vi "Auxiliary Association (Read).vi"(6 "ISOBUS address":T5=-1 caption="ISOBUS address (-1)", 8 "error in":errorcluster, 11 "Mercury Reference In":T2) -> (0 "error out":errorcluster, 2 "Auxiliary board UID":string, 3 "Mercury Reference Out":T2, 4 "Valid?":T1)   [LabVIEW 2014, in "Mercury iXX.lvlib" / "Control Loop.lvlib"]
doc: "Read the UID of the associated auxiliary board to the control loop."
uses:
  Control Loop.lvlib
  Controls/Mercury Reference.ctl
  Controls/Comms Transport Layer.ctl
  Private/Controls/Query Dynamic Reference.ctl
  Controls/ISOBus Address.ctl
  Controls/Is Valid LED.ctl
  Private/Controls/Command Verbs.ctl
  Mercury iXX.lvlib
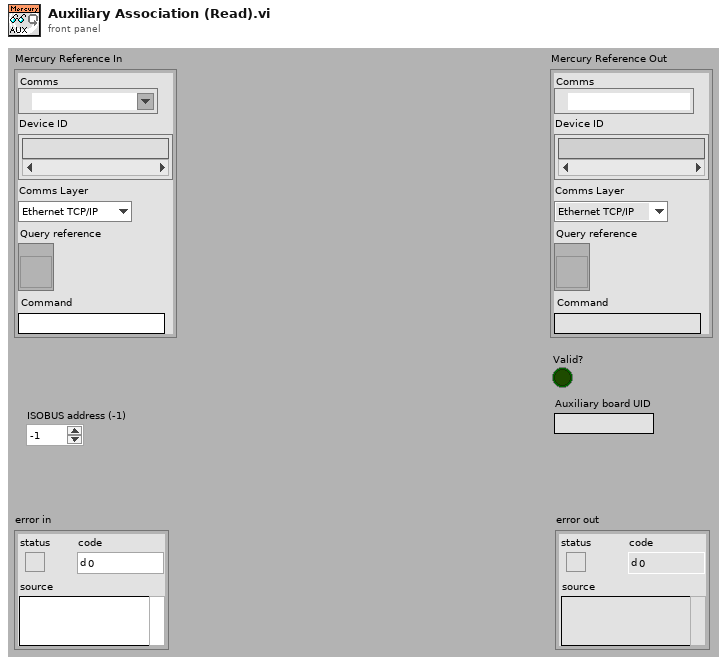
[diagram p1: front panel]
types:
  T1 = typedef "Mercury iXX.lvlib/Is Valid LED.ctl" = bool
  T2 = typedef "Mercury iXX.lvlib/Mercury Reference.ctl" = cluster{"Comms":refnum<visa-resource-name>, "Device ID":string[], "Comms Layer":T3, "Command":string, "Query reference":T4}
  T3 = typedef "Mercury iXX.lvlib/Comms Transport Layer.ctl" = enum16{"Ethernet TCP/IP", "USB", "ISOBus - RS-232", "GPIB"}
  T4 = typedef "Mercury iXX.lvlib/Query Dynamic Reference.ctl" = refnum<vi>
  T5 = typedef "Mercury iXX.lvlib/ISOBus Address.ctl" = i32
  T6 = typedef "Mercury iXX.lvlib/Command Verbs.ctl" = string
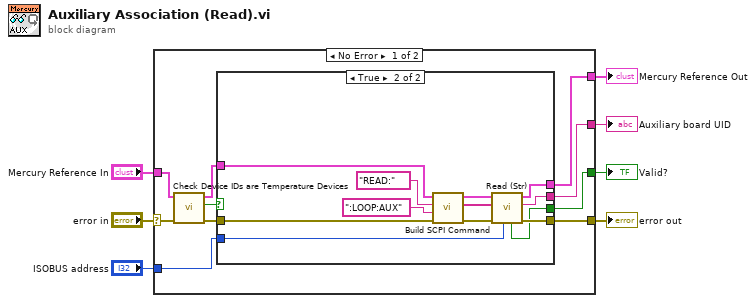
[diagram p0: block diagram]
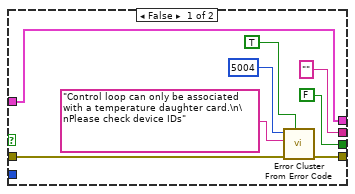
[diagram p2: hidden frame]
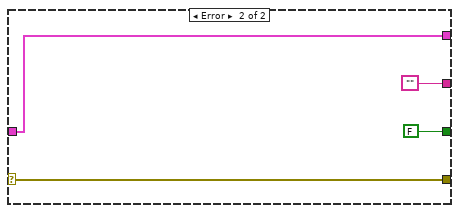
[diagram p3: hidden frame]
diagram:
  n1 = case shown="No Error" "error in" {
    selector: "error in" -> [w13 w41]
    tunnel: [w17 w38] -> w5
    tunnel: [w15 w41] -> w3
    tunnel: "ISOBUS address" -> [w16 _]
    tunnel: [w9 ""] -> w1
    tunnel: [w8 FALSE ("Valid?")] -> w2
    tunnel: "Mercury Reference In" -> [w11 w38]
    frame No Error {
      n2 = call "Check Device IDs are Temperature Devices.vi"("error in"=w13, "Mercury Reference In"=w11) -> ("error out"=w12:errorcluster, "Valid?"=w14:bool, "Mercury Reference Out"=w10:T2)  [unwired: 7 out]
      n3 = case shown="True" w14 {
        tunnel: w10 -> [w25 w33]
        tunnel: [w25 w29] -> w17
        tunnel: w12 -> [w23 w32]
        tunnel: w16 -> [_ w26]
        tunnel: [w24 w31] -> w15
        tunnel: ["" ("Response") w28] -> w9
        tunnel: [T1 FALSE ("Valid?") w27] -> w8
        frame False {
          n4 = call <vilib>:"Error Cluster From Error Code.vi"("show call chain? (False)"=TRUE, "error in (no error)"=w23, "error message (\"\")"="Control loop can only be associated with a temperature daughter card.\n\nPlease check device IDs" ("error message (\"\")"), "error code (0)"=5004) -> ("error out"=w24:errorcluster)  [unwired: 5 out]
        }
        frame True {
          n5 = call "Build SCPI Command.vi"("error in"=w32, "Noun(s)"=":LOOP:AUX" ("Command"), "Verb"=T6 "READ:", "Mercury Reference In"=w33) -> ("error out"=w30:errorcluster, "SCPI Message(s)"=w37:string[], "Mercury Reference Out"=w36:T2)  [unwired: 5 out]
          n6 = call "Read (Str).vi"("ISOBUS address"=w26, "error in"=w30, "SCPI Message(s)"=w37, "Mercury Reference In"=w36) -> ("error out"=w31:errorcluster, "Response"=w28:string, "Mercury Reference Out"=w29:T2, "Valid?"=w27:T1)  [unwired: 4 out]
        }
      }
    }
    frame Error {
    }
  }
  "Mercury Reference Out" <- w5
  "Auxiliary board UID" <- w1
  "error out" <- w3
  "Valid?" <- w2
